vi "UseCustomTimestamp.vi"(8 "error in (no error)":errorcluster, 9 "AcqSuccess":bool, 10 "CustomTimeStamp":dbl format="%.3f", 11 "BaseDriver in":refnum<class "BaseDriver.lvclass">) -> (0 "error out":errorcluster, 3 "BaseDriver out":refnum<class "BaseDriver.lvclass">)   [LabVIEW 2020, in "BaseDriver.lvclass"]
uses:
  BaseDriver.lvclass
  BaseDriver.lvclass/BaseDriver.ctl
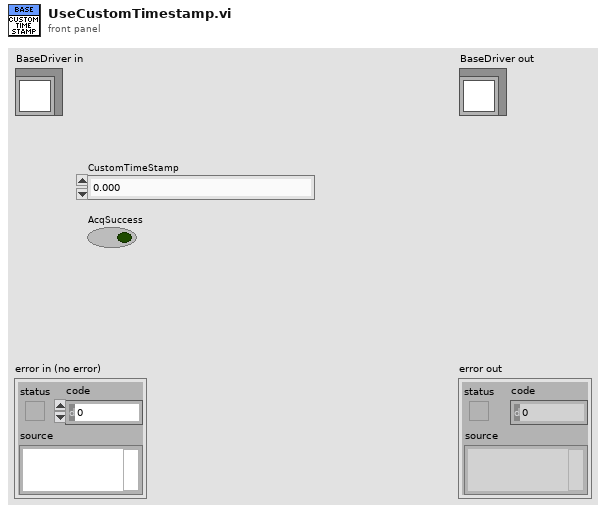
[diagram p1: front panel]
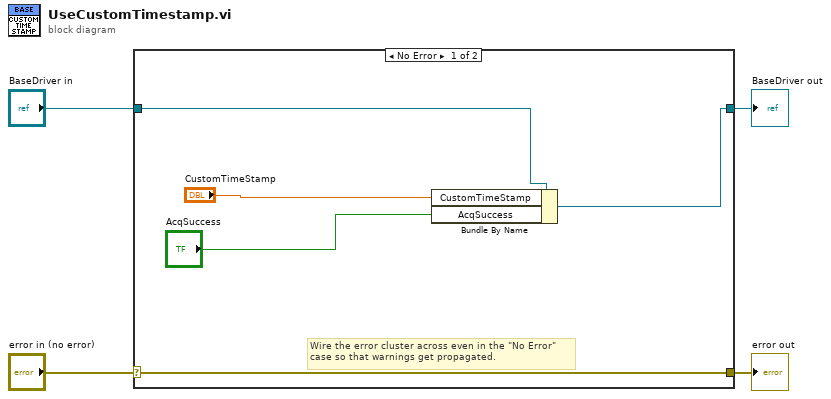
[diagram p0: block diagram]
diagram:
  n1 = case shown="No Error" "error in (no error)" {
    selector: "error in (no error)" -> [w9 w11]
    tunnel: [w9 w11] -> w3
    tunnel: [w6 w10] -> w1
    tunnel: "BaseDriver in" -> [w8 w10]
    frame No Error {
      # "Wire the error cluster across even in the \"No Error\"\ncase so that warnings get propagated."
      n2 = Bundle By Name(cluster=w8, "CustomTimeStamp"="CustomTimeStamp", "AcqSuccess"="AcqSuccess") -> (w6:refnum<class "BaseDriver.lvclass">)
    }
    frame Error {
    }
  }
  "error out" <- w3
  "BaseDriver out" <- w1
